vi "Begin-End.vi"(8 "Error In":errorcluster) -> (0 "Error Out":errorcluster)   [LabVIEW 2017, in "Tests.lvlib" / "Writer.lvlib"]
uses:
  Writer.lvlib
  src/LabPack/Public/Writer/Writer.lvclass/Writer.ctl
  src/LabPack/Public/Writer/Private/Handle Error.vi
  src/LabPack/Public/Writer/Public/Status/Read Is Error.vi
  src/LabPack/Public/Writer/Public/Status/Read Status.vi
  src/LabPack/Public/Writer/Public/Status/Read Status Message.vi
  src/LabPack/Public/Writer/Private/Begin by Value.vi
  src/LabPack/Public/Utility/Status Code.vi
  <vilib>/Utility/error.llb/Error Cluster From Error Code.vi
  src/LabPack/Public/Writer/Private/End by Value.vi
  src/LabPack/Public/Writer/Writer.lvclass
  <vilib>/addons/_JKI Toolkits/Caraya/classes/Test/Test.lvclass
  <vilib>/addons/_JKI Toolkits/Caraya/classes/Assert/Assert.lvclass
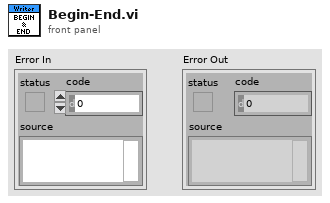
[diagram p1: front panel]
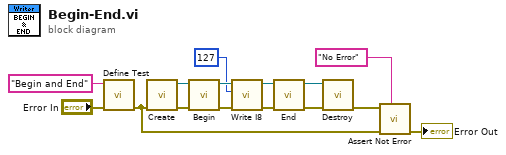
[diagram p0: block diagram]
diagram:
  n1 = call <vilib>:"Define Test.vi"("error in (no error)"="Error In", "Label (VI Title)"="Begin and End") -> ("error out"=w10:errorcluster)  [unwired: 9 in]
  n2 = call "Create.vi"("Error In"=w10) -> ("Error Out"=w8:errorcluster, "Writer"=w11:refnum<class "Writer.lvclass">)  [unwired: 9 in]
  n3 = call-poly "Begin.vi"("Error In"=w8, "Writer In"=w11) -> ("Error Out"=w6:errorcluster, "Writer Out"=w7:refnum<class "Writer.lvclass">)  [unwired: 8 in]
  n4 = call "Write I8.vi"("Error In"=w6, "Value"=i8 127, "Writer In"=w7) -> ("Error Out"=w4:errorcluster, "Writer Out"=w5:refnum<class "Writer.lvclass">)  [unwired: 7 in]
  n5 = call-poly "End.vi"("Error In"=w4, "Writer In"=w5) -> ("Error Out"=w2:errorcluster, "Writer Out"=w3:refnum<class "Writer.lvclass">)  [unwired: 7 in, 1 out]
  n6 = call "Destroy.vi"("Error In"=w2, "Writer"=w3) -> ("Error Out"=w9:errorcluster)  [unwired: 9 in]
  n7 = call <vilib>:"Assert Not Error.vi"("Label"="No Error", "error in (no error)"=w10, "Not Error?"=w9) -> ("error out"=→"Error Out":errorcluster)  [unwired: 8 in]
